vi "TCP Multiple Connections - Server.vi"() -> ()   [LabVIEW 2018]
doc: "This is the TCP server VI that supports multiple connections from client VIs."
uses:
  controls/TCP Multiple Connections State.ctl
  controls/TCP Multiple Connections Data.ctl
panel:
  out "192.168.1.104":bool
  out "Client Index":i32
  out "data out":string
  in  "Stop":bool
  out "# of Connections":i32
  # "Overview: Demonstrates the use of the TCP functions to initialize a TCP server that can send data to multiple client VIs.\nInstructions:\n1. Run the VI.\n2. Open TCP Multiple Connections - Client 1.vi and follow the instructions on its front panel.\n3. Open TCP Multiple Connections - Client 2.vi and follow the instructions on its front panel.\n4. Click Stop to stop the VI."
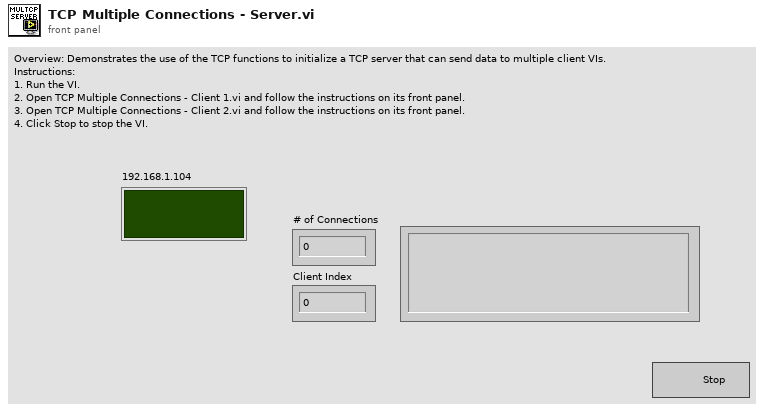
[diagram p1: front panel]
types:
  T1 = typedef "TCP Multiple Connections Data.ctl" = cluster{"Clients":refnum<k5>[], "Listener":refnum<k5>}
  T2 = typedef "TCP Multiple Connections State.ctl" = enum16{"Initialize", "Status Check", "Read Data", "Stop"}
  T3 = enum16{"Standard", "Buffered", "CRLF", "Immediate"}
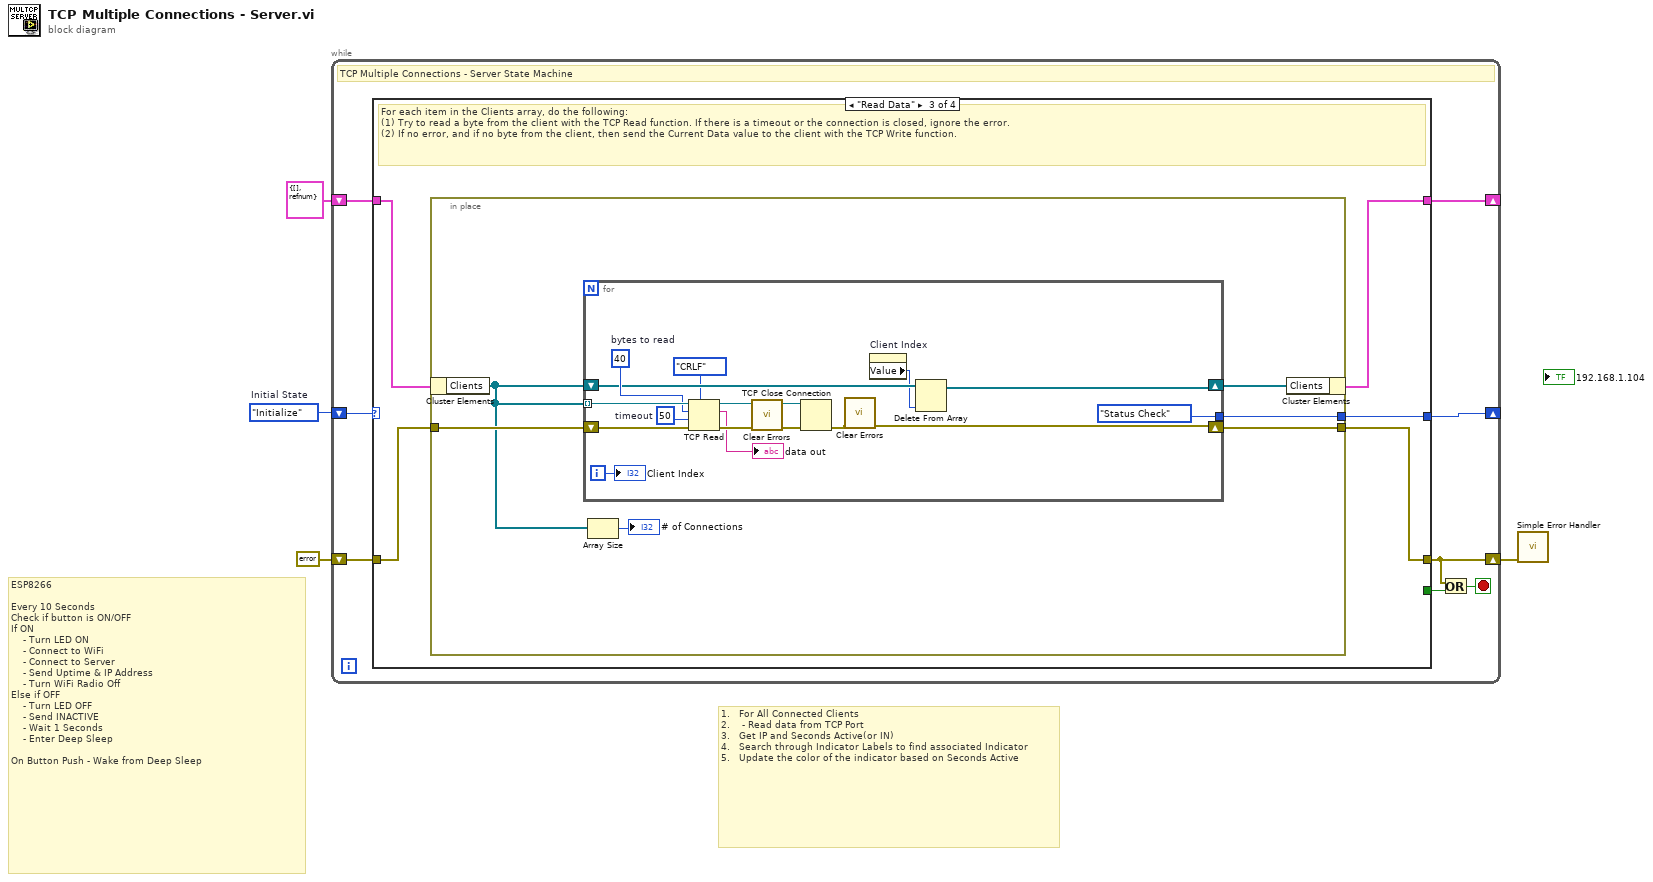
[diagram p0: block diagram]
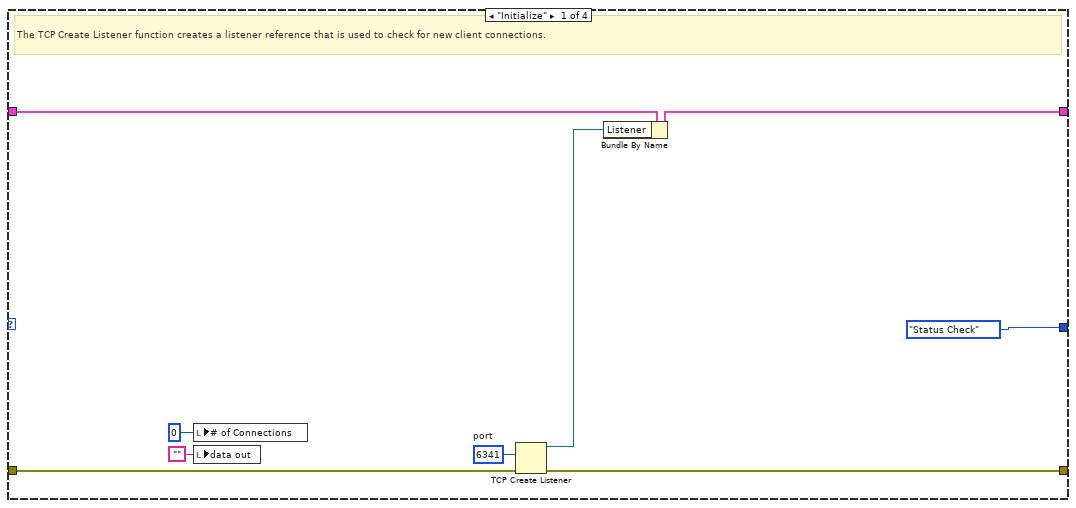
[diagram p2: hidden frame]
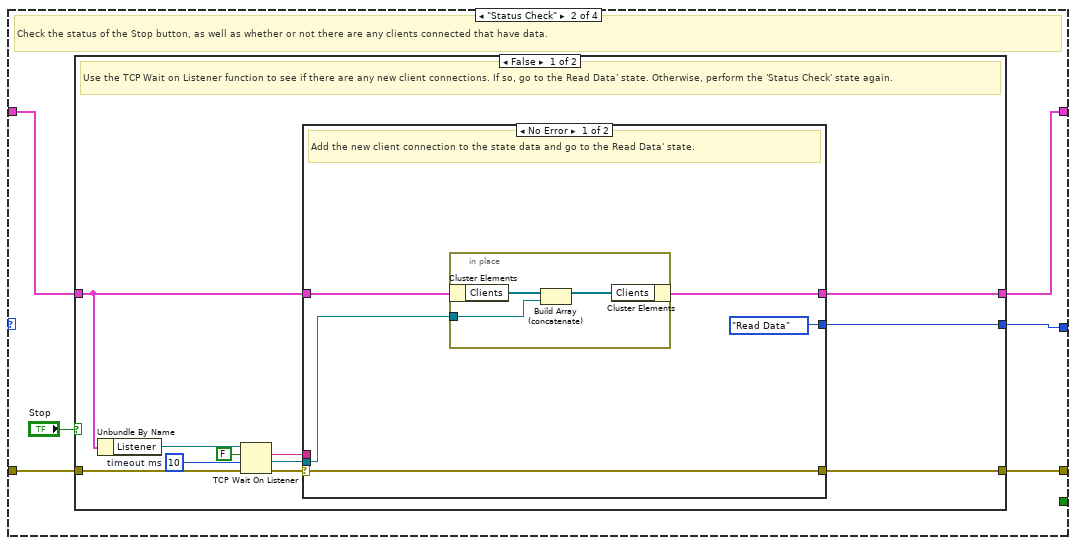
[diagram p3: hidden frame]
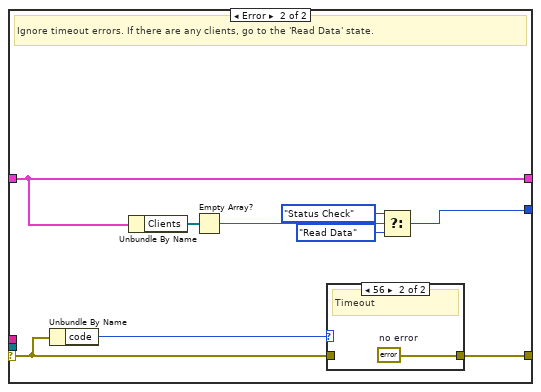
[diagram p4: hidden frame]
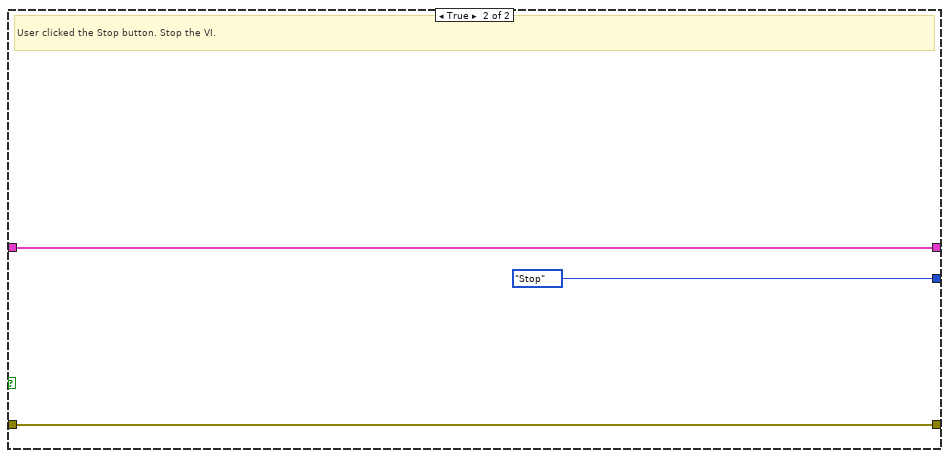
[diagram p6: hidden frame]
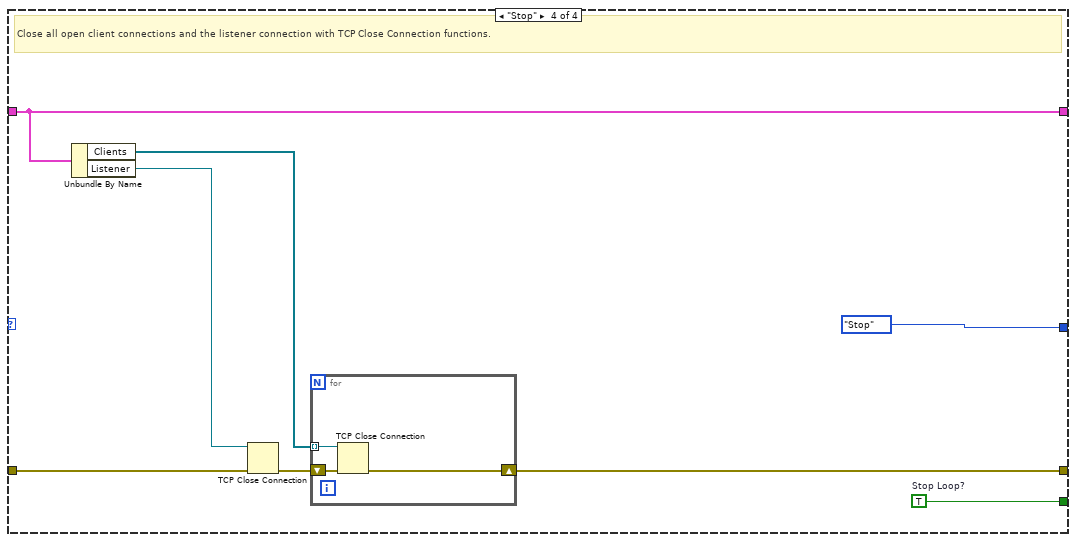
[diagram p7: hidden frame]
diagram:
  w4 = TCP_Multiple_Connections_State."Initialize"  # Initial State
  # "ESP8266\n\nEvery 10 Seconds\nCheck if button is ON/OFF\nIf ON\n    - Turn LED ON\n    - Connect to WiFi\n    - Connect to Server\n    - Send Uptime & IP Address\n    - Turn WiFi Radio Off\nElse if OFF\n    - Turn LED OFF\n    - Send INACTIVE\n    - Wait 1 Seconds\n    - Enter Deep Sleep\n\nOn Button Push - Wake from Deep Sleep"
  # "1.   For All Connected Clients\n2.    - Read data from TCP Port\n3.   Get IP and Seconds Active(or IN)\n4.   Search through Indicator Labels to find associated Indicator\n5.   Update the color of the indicator based on Seconds Active"
  n1 = while {
    shift-right: [w5] -> _
    shift-left: w4 -> [w12]
    shift-right: [w10] -> _
    shift-left: T1 {"Clients"=[], "Listener"=refnum} ("Data") -> [w11]
    shift-right: [w6] -> w1
    shift-left: errorcluster {"status"=FALSE, "code"=0, "source"=""} ("error constant") -> [w9]
    stop <- w7 stop-if-true
    # "TCP Multiple Connections - Server State Machine"
    n2 = case shown="\"Read Data\"" w12 {
      tunnel: [TCP_Multiple_Connections_State."Status Check" ("States") w27 w61 TCP_Multiple_Connections_State."Stop" ("(Value Not Used)")] -> w5
      tunnel: [_ _ _ w95] -> w8
      tunnel: w11 -> [w19 w23 w63 w94]
      tunnel: [w18 w22 w62 w94] -> w10
      tunnel: w9 -> [w21 w26 w65 w93]
      tunnel: [w20 w25 w64 w91] -> w6
      frame "Initialize" {
        w16 = u16 6341  # port
        # "The TCP Create Listener function creates a listener reference that is used to check for new client connections."
        n3 = local write "# of Connections"(0 ("Number of Client Connections")) -> ()
        n4 = local write "data out"("" ("data out")) -> ()
        n5 = TCP Create Listener(8:w21, 10:w16) -> (0:w20:errorcluster, 3:w17:refnum<k5>)  [unwired: 4 out]
        n6 = Bundle By Name(cluster=w19, "Listener"=w17) -> (w18:T1)
      }
      frame "Status Check" {
        # "Check the status of the Stop button, as well as whether or not there are any clients connected that have data."
        n7 = case shown="False" "Stop" {
          tunnel: [w38 TCP_Multiple_Connections_State."Stop" ("States")] -> w27
          tunnel: w26 -> [w37 w60]
          tunnel: [w30 w60] -> w25
          tunnel: w23 -> [w33 w59]
          tunnel: [w32 w59] -> w22
          frame False {
            w36 = 10  # timeout ms
            # "Use the TCP Wait on Listener function to see if there are any new client connections. If so, go to the Read Data' state. Otherwise, perform the 'Status Check' state again."
            n8 = Unbundle By Name(w33) -> ("Listener"=w31:refnum<k5>)
            n9 = TCP Wait On Listener(8:w37, 9:w36, 10:FALSE ("resolve remote address (T)"), 11:w31) -> (0:w35:errorcluster, 2:w29:string, 4:w34:refnum<k5>)  [unwired: 2 out]
            n10 = case shown="No Error" w35 {
              selector: w35 -> [w41 w55]
              tunnel: [TCP_Multiple_Connections_State."Read Data" ("Initial State") w49] -> w38
              tunnel: w34 -> [w42 _]
              tunnel: w33 -> [w43 w52]
              tunnel: [w40 w52] -> w32
              tunnel: [w41 w53] -> w30
              tunnel: w29 -> [_ _]
              frame No Error {
                # "Add the new client connection to the state data and go to the Read Data' state."
                n11 = in-place {
                  in-place-border: w42 -> [w44]
                  n12 = in-place-cluster #1(w43) -> ("Clients"=w46:refnum<k5>[])
                  n13 = Build Array (concatenate)(w46, w44) -> (w45:refnum<k5>[])
                  n14 = in-place-cluster #1("Clients"=w45) -> (w40:T1)
                }
              }
              frame Error {
                # "Ignore timeout errors. If there are any clients, go to the 'Read Data' state."
                n15 = Unbundle By Name(w55) -> ("code"=w54:i32)
                n16 = Unbundle By Name(w52) -> ("Clients"=w51:refnum<k5>[])
                n17 = Empty Array?(array=w51) -> (empty?=w50:bool)
                n18 = case shown="56" w54 {
                  tunnel: w55 -> [w56 _]
                  tunnel: [w56 w57] -> w53
                  frame Default {
                  }
                  frame 56 {
                    w57 = errorcluster {"status"=FALSE, "code"=0, "source"=""}  # no error
                    # "Timeout"
                  }
                }
                n19 = Select(t=TCP_Multiple_Connections_State."Status Check" ("States"), s=w50, f=TCP_Multiple_Connections_State."Read Data" ("Initial State")) -> (s? t:f=w49:T2)
              }
            }
          }
          frame True {
            # "User clicked the Stop button. Stop the VI."
          }
        }
      }
      frame "Read Data" {
        # "For each item in the Clients array, do the following:\n(1) Try to read a byte from the client with the TCP Read function. If there is a timeout or the connection is closed, ignore the error. \n(2) If no error, and if no byte from the client, then send the Current Data value to the client with the TCP Write function."
        n20 = in-place {
          in-place-border: w65 -> [w71]
          in-place-border: [w70] -> w64
          in-place-border: [w68] -> w61
          n21 = in-place-cluster #2(w63) -> ("Clients"=w66:refnum<k5>[])
          n22 = for {
            tunnel: w66 -> [w87] mode=indexing
            shift-right: [w83] -> w70
            shift-left: w71 -> [w85]
            tunnel: [TCP_Multiple_Connections_State."Status Check" ("States")] -> w68
            shift-right: [w78] -> w67
            shift-left: w66 -> [w77]
            i -> [w73]
            w86 = 50  # timeout
            w82 = 40  # bytes to read
            n23 = TCP Read(connection ID=w87, bytes to read=w82, error in (no error)=w85, 7:T3."CRLF" ("mode (standard)"), 9:w86) -> (connection ID out=w84:refnum<k5>, data out=→"data out":string, error out=w81:errorcluster)
            n24 = call <vilib>:"Clear Errors.vi"("error in (no error)"=w81) -> ("error out"=w76:errorcluster)  [unwired: 5 in, 1 out]
            n25 = TCP Close Connection(connection ID=w84, error in (no error)=w76) -> (error out=w74:errorcluster)  [unwired: 1 in, 1 out]
            n26 = call <vilib>:"Clear Errors.vi"("error in (no error)"=w74) -> ("error out"=w83:errorcluster)  [unwired: 5 in, 1 out]
            n27 = property on="Client Index" class="DigNum (strict)"() -> ("Value"=w75:i32)  [unwired: 2 in, 2 out]
            n28 = Delete From Array(array=w77, index=w75) -> (array with subset deleted=w78:refnum<k5>[])  [unwired: 1 in, 1 out]
            "Client Index" <- w73
          }
          n29 = Array Size(array=w66) -> (size(s)=→"# of Connections":i32)
          n30 = in-place-cluster #2("Clients"=w67) -> (w62:T1)
        }
      }
      frame "Stop" {
        w95 = TRUE  # Stop Loop?
        # "Close all open client connections and the listener connection with TCP Close Connection functions."
        n31 = Unbundle By Name(w94) -> ("Clients"=w92:refnum<k5>[], "Listener"=w89:refnum<k5>)
        n32 = TCP Close Connection(connection ID=w89, error in (no error)=w93) -> (error out=w90:errorcluster)  [unwired: 1 in, 1 out]
        n33 = for {
          shift-right: [w97] -> w91
          shift-left: w90 -> [w98]
          tunnel: w92 -> [w96] mode=indexing
          n34 = TCP Close Connection(connection ID=w96, error in (no error)=w98) -> (error out=w97:errorcluster)  [unwired: 1 in, 1 out]
        }
      }
    }
    n35 = Or(x=w6, y=w8) -> (x .or. y?=w7:bool)
  }
  n36 = call <vilib>:"Simple Error Handler.vi"("error in (no error)"=w1) -> ()  [unwired: 4 in, 5 out]
